vi "Stop Core.vi"(10 "final error code":i32, 11 "LF2R IDE in":refnum<class "LF2R IDE.lvclass">) -> (3 "LF2R IDE out":refnum<class "LF2R IDE.lvclass">)   [LabVIEW 2018, in "LF2R IDE.lvlib" / "LF2R IDE.lvclass"]
doc: "In addition to the following, this method also sends a message to the monitor to notify it that the actor has stopped execution.\n\n(<B>Filename</B>: Actor Framework.lvlib:Actor.lvclass:Stop Core.vi)\n\nDefines what the actor does before it stops. Use the <B>final error code</B> input to determine whether the actor shut down in response to an error.\n\nBy default, this method does nothing. A descendant class may override it to define behavior, such as shutting down any processes the actor initiated in its override of the Actor Core method.\n\nCopyright: MGI\n\nAuthored by Derek Trepanier\nsupport@mooregoodideas.com\nwww.mooregoodideas.com\n\nCopyright (c) 2014, Moore Good Ideas, Inc.\n\nAll rights reserved.\n\nRedistribution and use in source and binary forms, with or without modification, are permitted provided that the following conditions are met:\n\n * Redistributions of source code must retain the above copyright notice, this list of conditions and the following disclaimer.\n * Redistributions in binary form must reproduce the above copyright notice, this list of conditions and the following disclaimer in the documentation and/or other materials provided with the distribution.\n * Neither the name of Moore Good Ideas, Inc. nor the names of its contributors may be used to endorse or promote products derived from this software without specific prior written permission.\n\nTHIS SOFTWARE IS PROVIDED BY THE COPYRIGHT HOLDERS AND CONTRIBUTORS \"AS IS\" AND ANY EXPRESS OR IMPLIED WARRANTIES, INCLUDING, BUT NOT LIMITED TO, THE IMPLIED WARRANTIES OF MERCHANTABILITY AND FITNESS FOR A PARTICULAR PURPOSE ARE DISCLAIMED. IN NO EVENT SHALL THE COPYRIGHT OWNER OR CONTRIBUTORS BE LIABLE FOR ANY DIRECT, INDIRECT, INCIDENTAL, SPECIAL, EXEMPLARY, OR CONSEQUENTIAL DAMAGES (INCLUDING, BUT NOT LIMITED TO, PROCUREMENT OF SUBSTITUTE GOODS OR SERVICES; LOSS OF USE, DATA, OR PROFITS; OR BUSINESS INTERRUPTION) HOWEVER CAUSED AND ON ANY THEORY OF LIABILITY, WHETHER IN CONTRACT, STRICT LIABILITY, OR TORT (INCLUDING NEGLIGENCE OR OTHERWISE) ARISING IN ANY WAY OUT OF THE USE OF THIS SOFTWARE, EVEN IF ADVISED OF THE POSSIBILITY OF SUCH DAMAGE."
uses:
  LF2R IDE.lvclass
  LF2R IDE.lvclass/LF2R IDE.ctl
  <vilib>/MGI/Panel Manager/Panel Actor/Panel Actor/Panel Actor.lvclass
  <userlib>/_MGI/Menu Building/MenuTypes/Vi/MGI_VI.lvclass
  ScintillaNET/ScintillaNET.lvclass
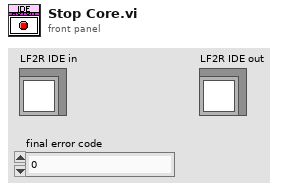
[diagram p1: front panel]
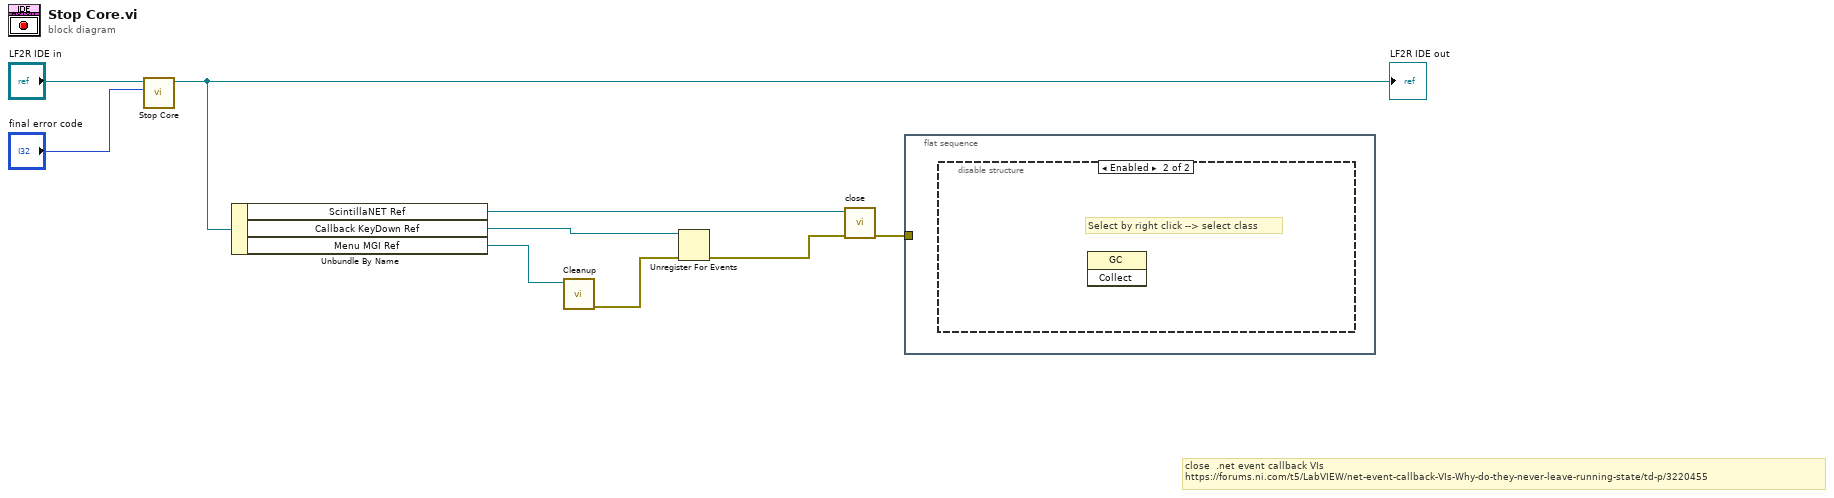
[diagram p0: block diagram]
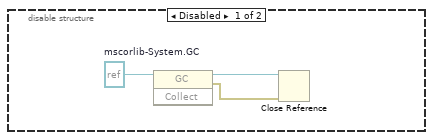
[diagram p2: hidden frame]
diagram:
  # "close  .net event callback VIs \nhttps://forums.ni.com/t5/LabVIEW/net-event-callback-VIs-Why-do-they-never-leave-running-state/td-p/3220455"
  n1 = call-parent "Stop Core.vi"("final error code"="final error code", "Monitored Actor in"="LF2R IDE in") -> ("Monitored Actor out"=w7:refnum<class "LF2R IDE.lvclass">)  [unwired: 9 in]
  "LF2R IDE out" <- w7
  n2 = Unbundle By Name(w7) -> ("ScintillaNET Ref"=w6:refnum<class "ScintillaNET.lvclass">, "Callback KeyDown Ref"=w4:refnum<k27>, "Menu MGI Ref"=w3:refnum<class "MGI_VI.lvclass">)
  n3 = call-dynamic "Cleanup.vi"("VI"=w3) -> ("error out"=w1:errorcluster)  [unwired: 10 in]
  n4 = Unregister For Events(event registration refnum=w4, error in=w1) -> (error out=w5:errorcluster)
  n5 = call "close.vi"("error in (no error)"=w5, "ScintillaNET in"=w6) -> ("error out"=w2:errorcluster)  [unwired: 9 in]
  n6 = flat-sequence {
    tunnel: w2 -> [_]
    frame #0 {
      n7 = disable-structure shown="Enabled" {
        frame Disabled {
          w12 = refnum<k24> refnum  # mscorlib-System.GC
          n8 = invoke class="GC" method="Collect"(reference=w12) -> (reference out=w11:refnum<k24>, error out=w10:errorcluster)  [unwired: 2 in, 1 out]
          n9 = Close Reference(reference=w11, error in (no error)=w10) -> ()  [unwired: 1 out]
        }
        frame Enabled {
          # "Select by right click --> select class"
          n10 = invoke class="GC" method="Collect"() -> ()  [unwired: 3 in, 3 out]
        }
      }
    }
  }
